vi "Load Antidoc Project Toolkit.vi"(8 "error in":errorcluster, 9 "Document Title":string, 10 "Project Path":path, 11 "Config":refnum<class "Config.lvclass">) -> (0 "error out":errorcluster, 3 "Config out":refnum<class "Lv Proj Config.lvclass">)   [LabVIEW 2020, in "CICD.lvlib"]
uses:
  CICD.lvlib
  <vilib>/Wovalab/AntiDoc/Document Type/Add-ons/LabVIEW Project/Lv Proj Config/Lv Proj Config.lvclass
  <vilib>/Wovalab/AntiDoc/Document Type/Config/Config.lvclass
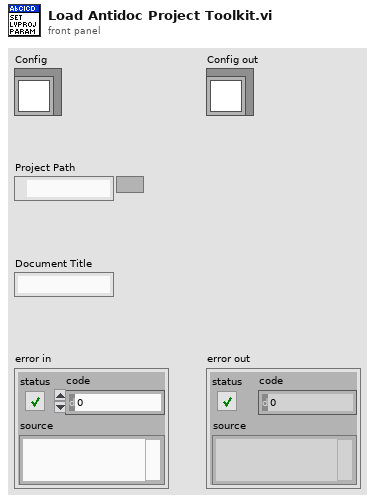
[diagram p1: front panel]
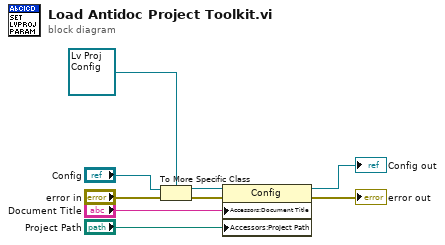
[diagram p0: block diagram]
diagram:
  n1 = To More Specific Class(target class=refnum<class "Lv Proj Config.lvclass"> refnum, reference="Config", error in="error in") -> (specific class reference=w5:refnum<class "Lv Proj Config.lvclass">, error out=w8:errorcluster)
  n2 = property class="Config"(reference=w5, error in=w8, "Accessors:Document Title"="Document Title", "Accessors:Project Path"="Project Path") -> (reference out=→"Config out":refnum<class "Lv Proj Config.lvclass">, error out=→"error out":errorcluster)
